vi "programa11.vi"() -> ()   [LabVIEW 2011]
uses:
  <vilib>/express/express arith-compare/Formula/XNode/ExpressFormulaBlockNode.xnode
panel:
  out "Contador":dbl
  out "Par":bool
  out "Impar":bool
  out "Contador impares":dbl
  out "Contador pares":dbl
  out "Numero":dbl
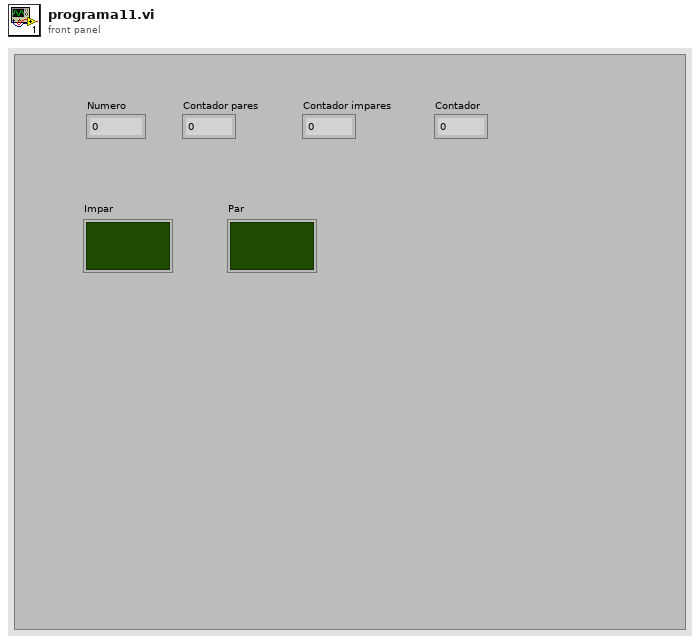
[diagram p1: front panel]
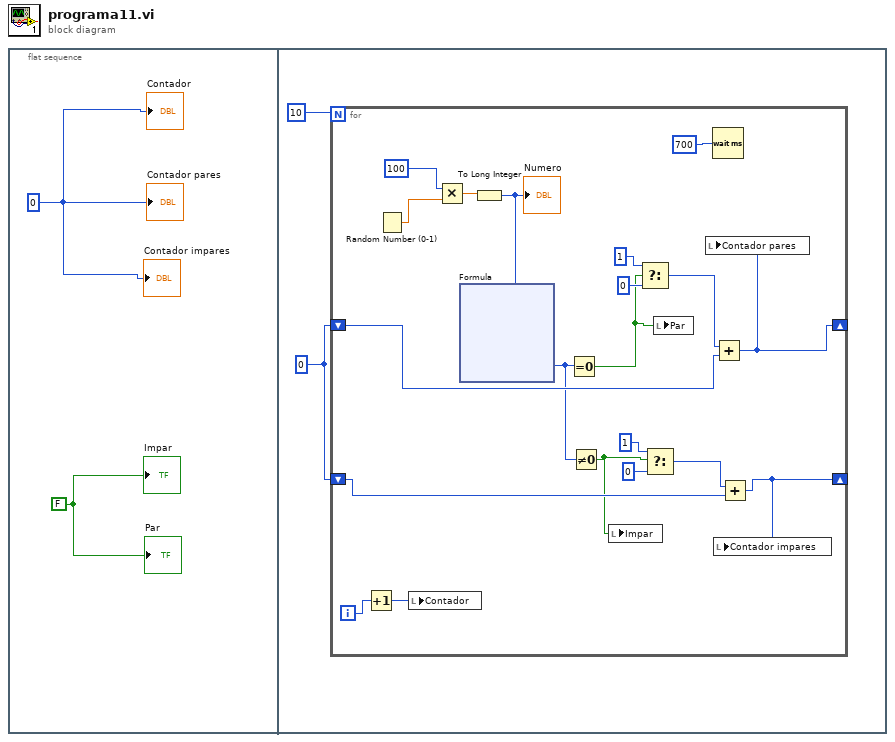
[diagram p0: block diagram]
diagram:
  n1 = flat-sequence {
    frame #0 {
      w1 = FALSE
      w2 = 0
      "Impar" <- w1
      "Par" <- w1
      "Contador" <- w2
      "Contador pares" <- w2
      "Contador impares" <- w2
    }
    frame #1 {
      w3 = 0
      n2 = for {
        N: 10 -> [_]
        shift-right: [w16] -> _
        shift-left: w3 -> [w17]
        shift-right: [w10] -> _
        shift-left: w3 -> [w12]
        i -> [w6]
        n3 = Increment(x=w6) -> (x+1=w5:i32)
        n4 = Random Number (0-1)() -> (number: 0 to 1=w23:dbl)
        n5 = local write "Contador"(w5) -> ()
        n6 = Multiply(x=100, y=w23) -> (x*y=w22:dbl)
        n7 = To Long Integer(number=w22) -> (32bit integer=w21:i32)
        "Numero" <- w21
        n8 = xnode "Formula"("X1"=w21) -> ("Result"=w15:i32)  [unwired: 1 in, 1 out]
        n9 = Equal To 0?(x=w15) -> (x = 0?=w8:bool)
        n10 = Not Equal To 0?(x=w15) -> (x != 0?=w9:bool)
        n11 = local write "Impar"(w9) -> ()
        n12 = Select(t=1, s=w8, f=0) -> (s? t:f=w18:i32)
        n13 = Select(t=1, s=w9, f=0) -> (s? t:f=w11:i32)
        n14 = local write "Par"(w8) -> ()
        n15 = Wait (ms)(milliseconds to wait=700) -> ()  [unwired: 1 out]
        n16 = Add(x=w18, y=w17) -> (x+y=w16:i32)
        n17 = local write "Contador pares"(w16) -> ()
        n18 = Add(x=w11, y=w12) -> (x+y=w10:i32)
        n19 = local write "Contador impares"(w10) -> ()
      }
    }
  }
